vi "Traffic Light.vi"() -> ()   [LabVIEW 2023]
panel:
  in  "stop":bool
  out "green":bool
  out "yellow":bool
  out "red":bool
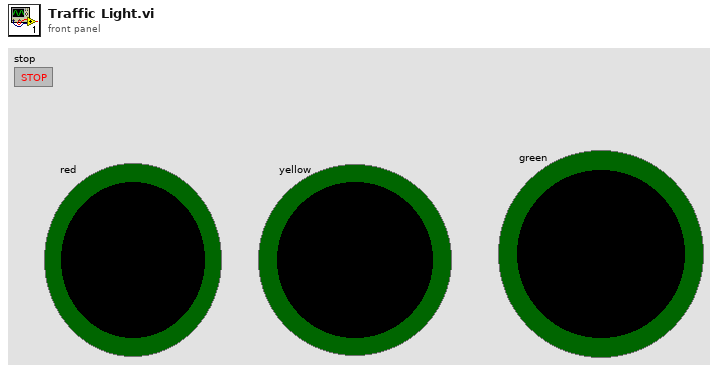
[diagram p1: front panel]
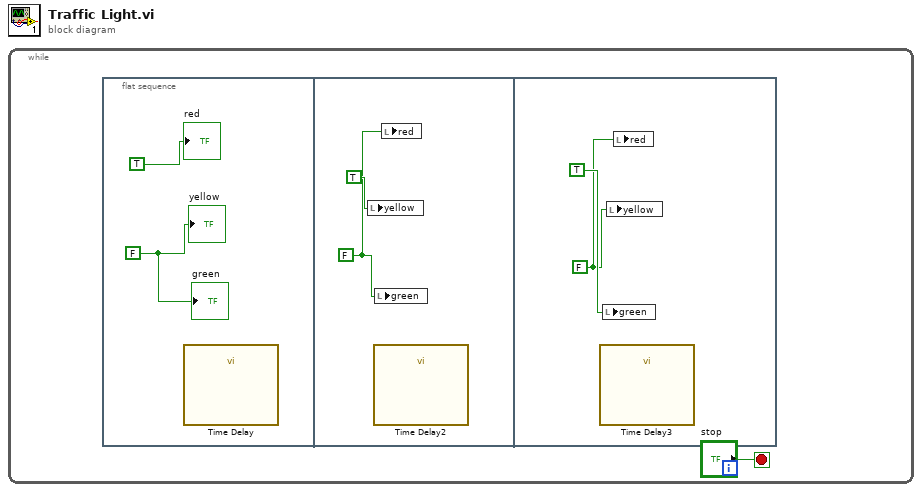
[diagram p0: block diagram]
diagram:
  n1 = while {
    stop <- "stop" stop-if-true
    n2 = flat-sequence {
      frame #0 {
        w2 = FALSE
        n3 = call "Time Delay"() -> ()  [unwired: 11 in, 1 out]
        "red" <- TRUE
        "yellow" <- w2
        "green" <- w2
      }
      frame #1 {
        w4 = FALSE
        n4 = local write "yellow"(TRUE) -> ()
        n5 = call "Time Delay2"() -> ()  [unwired: 11 in, 1 out]
        n6 = local write "green"(w4) -> ()
        n7 = local write "red"(w4) -> ()
      }
      frame #2 {
        w6 = FALSE
        n8 = call "Time Delay3"() -> ()  [unwired: 11 in, 1 out]
        n9 = local write "green"(TRUE) -> ()
        n10 = local write "yellow"(w6) -> ()
        n11 = local write "red"(w6) -> ()
      }
    }
  }
